vi "SVL Close Waterfall Display.vi"(0 "waterfall ref":refnum<vi>, 11 "error in (no error)":errorcluster) -> (15 "error out":errorcluster)   [LabVIEW 2017]
doc: "Closes the waterfall display specified by <B>waterfall ref</B>."
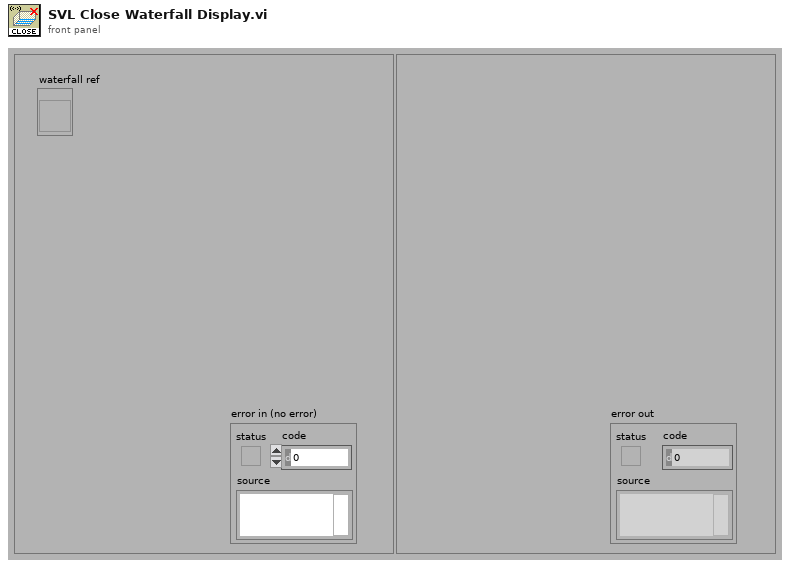
[diagram p1: front panel]
types:
  T1 = enum32{"Bad", "Idle", "Run top level", "Running"}
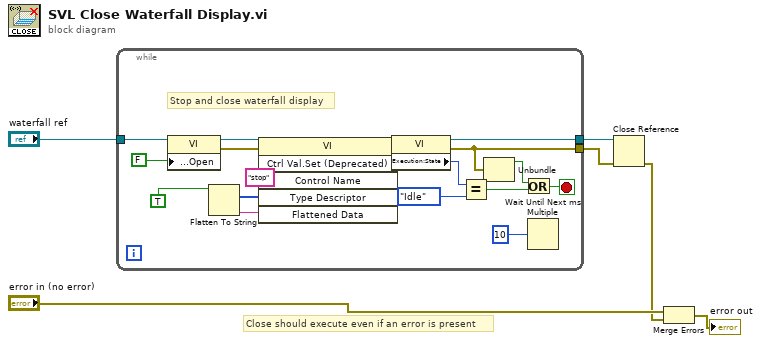
[diagram p0: block diagram]
diagram:
  # "Close should execute even if an error is present"
  n1 = while {
    tunnel: [w14] -> w4
    tunnel: [w9] -> w5
    tunnel: "waterfall ref" -> [w20]
    stop <- w7 stop-if-true
    # "Stop and close waterfall display"
    n2 = property class="VI"(reference=w20, "Front Panel Window:Open"=FALSE ("Front Panel.Open")) -> (reference out=w21:refnum<vi>, error out=w19:errorcluster)  [unwired: 1 in]
    n3 = Flatten To String(anything=TRUE ("Front Panel.Open")) -> (data string=w22:string, type string=w23:i16[])  [unwired: 3 in, 1 out]
    n4 = invoke class="VI" method="Ctrl Val.Set (Deprecated)"(reference=w21, error in=w19, "Control Name"="stop", "Type Descriptor"=w23, "Flattened Data"=w22) -> (reference out=w16:refnum<vi>, error out=w15:errorcluster)  [unwired: 1 in, 4 out]
    n5 = property class="VI"(reference=w16, error in=w15) -> (reference out=w14:refnum<vi>, error out=w9:errorcluster, "Execution:State"=w13:T1)
    n6 = Equal?(x=w13, y=T1."Idle") -> (x = y?=w10:bool)
    n7 = Unbundle(w9) -> ("status"=w8:bool)  [unwired: 2 out]
    n8 = Or(x=w8, y=w10) -> (x .or. y?=w7:bool)
    n9 = Wait Until Next ms Multiple(millisecond multiple=u32 10) -> ()  [unwired: 1 out]
  }
  n10 = Close Reference(reference=w4, error in (no error)=w5) -> (error out=w2:errorcluster)
  n11 = Merge Errors("error in (no error)", w2) -> (→"error out":errorcluster)
